vi "Initiate.vi"(8 "error in (no error)":errorcluster, 10 "Mode (0:Arm)":u16(ring) items=["Arm", "Force Trigger"], 11 "VISA resource name":refnum<visa-resource-name>) -> (0 "error out":errorcluster, 3 "VISA resource name out":refnum<visa-resource-name>)   [LabVIEW 2013, in "LeCroy Wave Series.lvlib"]
doc: "Initiates a waveform acquisition. After you call this VI, the instrument leaves the Idle state and waits for a trigger.\n\n<B>Note</B> This VI does not check the instrument status. Typically, you call this VI only in a sequence of calls to other low-level instrument driver VIs. The sequence performs one operation. You use the low-level VIs to optimize one or more aspects of interaction with the instrument."
uses:
  LeCroy Wave Series.lvlib
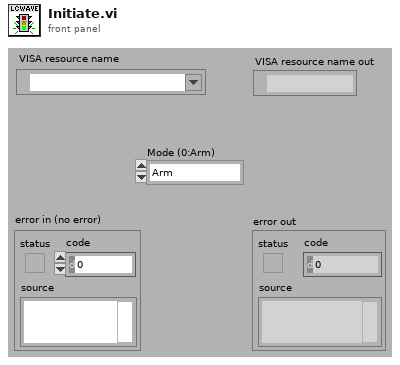
[diagram p1: front panel]
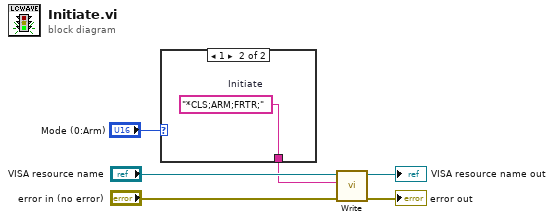
[diagram p0: block diagram]
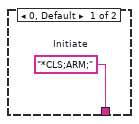
[diagram p2: hidden frame]
diagram:
  n1 = case shown="1" "Mode (0:Arm)" {
    tunnel: [w7 w8] -> w1
    frame 0, Default {
      w7 = "*CLS;ARM;"  # Initiate
    }
    frame 1 {
      w8 = "*CLS;ARM;FRTR;"  # Initiate
    }
  }
  n2 = call "Write.vi"("error in (no error)"="error in (no error)", "Write Buffer"=w1, "VISA resource name"="VISA resource name") -> ("error out"=→"error out":errorcluster, "VISA resource name out"=→"VISA resource name out":refnum<visa-resource-name>)  [unwired: 6 in, 1 out]
